vi "Spawn Child placeholder.vi"(7 "Actor in":refnum<class "Actor.lvclass">) -> (0 "Error out":errorcluster, 5 "Actor out":refnum<class "Actor.lvclass">)   [LabVIEW 2025, in "_Template.lvlib" / "Templates.lvlib" / "TEMPLATE jettl Actor.lvlib" / "TEMPLATE Actor.lvlib"]
uses:
  TEMPLATE Actor.lvlib
  jettl/jettl/Actor/Actor.lvclass
  Static Child UIDs.ctl
  Init Actor.vi
  jettl/jettl/jettl.lvlib
  TEMPLATE jettl Actor.lvlib
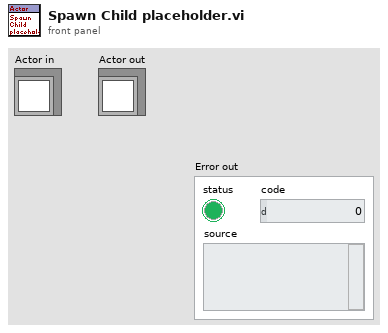
[diagram p1: front panel]
types:
  T1 = typedef "_Template.lvlib/Templates.lvlib/TEMPLATE jettl Actor.lvlib/TEMPLATE Actor.lvlib/Static Child UIDs.ctl" = enum16{"placeholder"}
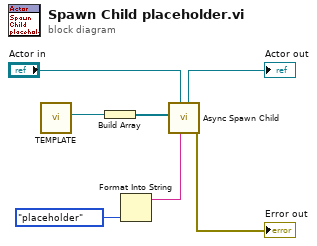
[diagram p0: block diagram]
diagram:
  n1 = call-poly "TEMPLATE.vi"() -> ("Actor"=w1:refnum<class "Actor.lvclass">)  [unwired: 11 in]
  n2 = Build Array(w1) -> (w5:refnum<class "Actor.lvclass">[])
  n3 = Format Into String(Static_Child_UIDs."placeholder" ("Static Child UIDs")) -> (resulting string=w4:string)  [unwired: 3 in, 1 out]
  n4 = call "Async Spawn Child.vi"("UID"=w4, "Actor in"="Actor in", "Local Layers"=w5) -> ("Error out"=→"Error out":errorcluster, "Actor out"=→"Actor out":refnum<class "Actor.lvclass">)  [unwired: 7 in]
